vi "LVClass_SlopesPostProcessList AddSlopesPostProcessorList.vi"(0 "SlopesPostProcessorList in":refnum<class "SlopesPostProcessorList.lvclass">, 5 "Position":u32, 7 "SlopesPostProcessorList to add":refnum<class "SlopesPostProcessorList.lvclass">, 11 "error in (no error)":errorcluster) -> (4 "SlopesPostProcessorList out":refnum<class "SlopesPostProcessorList.lvclass">, 15 "error out":errorcluster)   [LabVIEW 2020, in "SlopesPostProcessorList.lvclass"]
doc: "Insert a SlopesPostProcessorList SubSlopesPostProcessorList in the\nSlopesPostProcessorList.\n\n--------------------------------------------------------------------------------\n\n<B>SlopesPostProcessorListIn </B> : SlopesPostProcessorList object.\n<B>SlopesPostProcessorListOut </B> : SlopesPostProcessorList object.\n<B>position </B> : Position of the processor in the SlopesPostProcessorList.\n<B>SubSlopesPostProcessorList </B> : SlopesPostProcessorList object.\n<B>ErrorIn </B> : Error\n<B>ErrorOut </B> : Error\n\n--------------------------------------------------------------------------------"
uses:
  SlopesPostProcessorList.lvclass
  SlopesPostProcessorList.lvclass/SlopesPostProcessorList.ctl
  LVClass_SlopesPostProcessList Read SlopesPostProccessor.vi
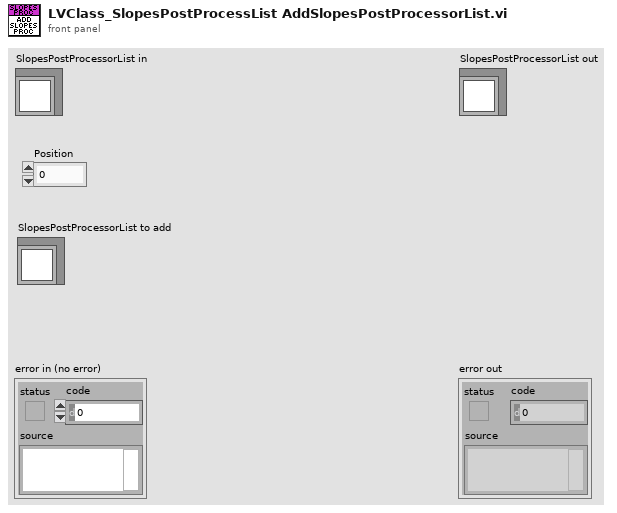
[diagram p1: front panel]
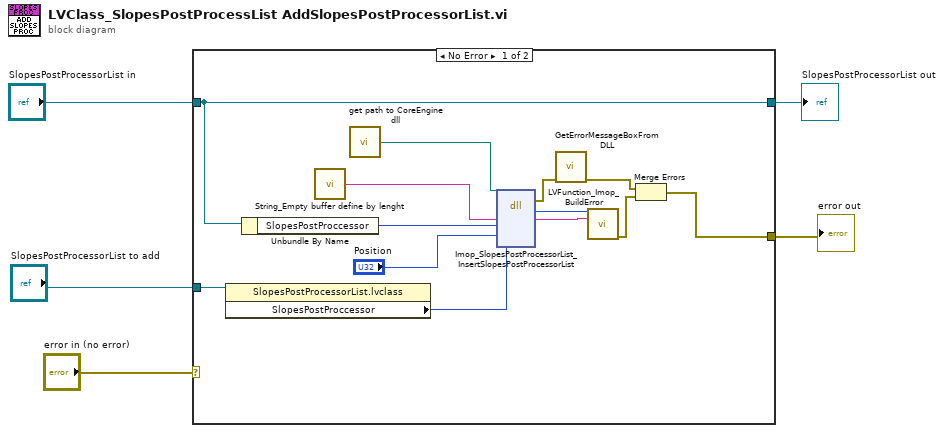
[diagram p0: block diagram]
diagram:
  n1 = case shown="No Error" "error in (no error)" {
    selector: "error in (no error)" -> [_ w19]
    tunnel: "SlopesPostProcessorList in" -> [w10 w20]
    tunnel: [w10 w20] -> w3
    tunnel: [w6 w19] -> w2
    tunnel: "SlopesPostProcessorList to add" -> [w13 _]
    frame No Error {
      n2 = property class="SlopesPostProcessorList.lvclass"(reference=w13) -> ("SlopesPostProccessor"=w12:i32)  [unwired: 1 in, 2 out]
      n3 = Unbundle By Name(w10) -> ("SlopesPostProccessor"=w9:i32)
      n4 = call "String_Empty buffer define by lenght.vi"() -> ("Empty buffer"=w18:string)  [unwired: 1 in]
      n5 = call "get path to CoreEngine dll.vi"() -> ("path to c_interface_vc100.dll"=w15:path)  [unwired: 12 in, 3 out]
      n6 = dll-call lib="D:/soft/HASO_v3/SVN_trunk/ImOpCoreEngine4_LV2011/DLLs/c_interface_vc100.dll" fn="Imop_SlopesPostProcessorList_InsertSlopesPostProcessorList"(path in=w15, "message"=w18, "objet"=w9, "Position"="Position", "SlopesPostProcessorList"=w12) -> (error out=w14:errorcluster, "return type"=w16:i32, "message"=w17:string)  [unwired: 5 in, 1 out]
      n7 = call "GetErrorMessageBoxFromDLL.vi"("error IN"=w14) -> ("error OUT"=w8:errorcluster)  [unwired: 10 in]
      n8 = call "LVFunction_Imop_BuildError.vi"("code"=w16, "String to Prepend to source (\"\")"=w17) -> ("error out"=w7:errorcluster)  [unwired: 13 in]
      n9 = Merge Errors(w8, w7) -> (w6:errorcluster)
    }
    frame Error {
    }
  }
  "error out" <- w2
  "SlopesPostProcessorList out" <- w3
